vi "rigol-dg1000.vi"() -> ()   [LabVIEW 2024]
uses:
  <vilib>/Instr/_visa.llb/VISA Open Access Mode.ctl
  <vilib>/measure/NI_MABase.lvlib
panel:
  out "Ch2 Freq":dbl caption="output 1" format="%#_6pHz"
  out "CH2 Volt":dbl caption="output 1" format="%#_6pVpp"
  out "CH2 status":bool
  out "Waveform CH2":waveform(dbl)(graph)
  out "Waveform CH1":waveform(dbl)(graph)
  out "CH1 status":bool
  out "CH1 Volt":dbl caption="output 1" format="%#_6pVpp"
  out "Ch1 Freq":dbl caption="output 1" format="%#_6pHz"
  in  "stop":bool
  out "error out":errorcluster
  in  "error in (no error)":errorcluster
  in  "VISA resource name":refnum<visa-resource-name>="TCPIP0::172.16.15.122::inst0::INSTR"
  # "CH1"
  # "CH2"
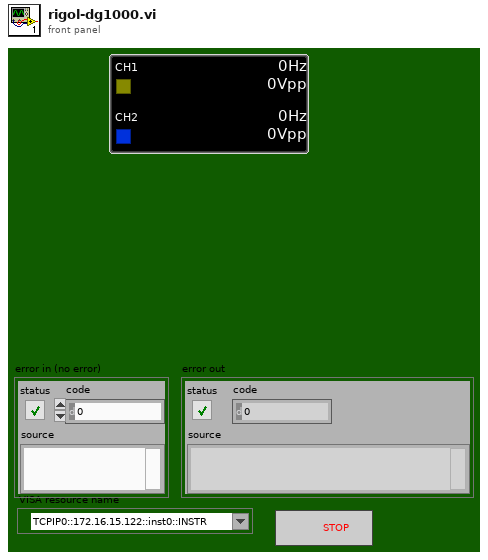
[diagram p1: front panel]
types:
  T1 = typedef "VISA Open Access Mode.ctl" = u32
  T2 = enum16{"Sine Wave", "Triangle Wave", "Square Wave", "Sawtooth Wave"}
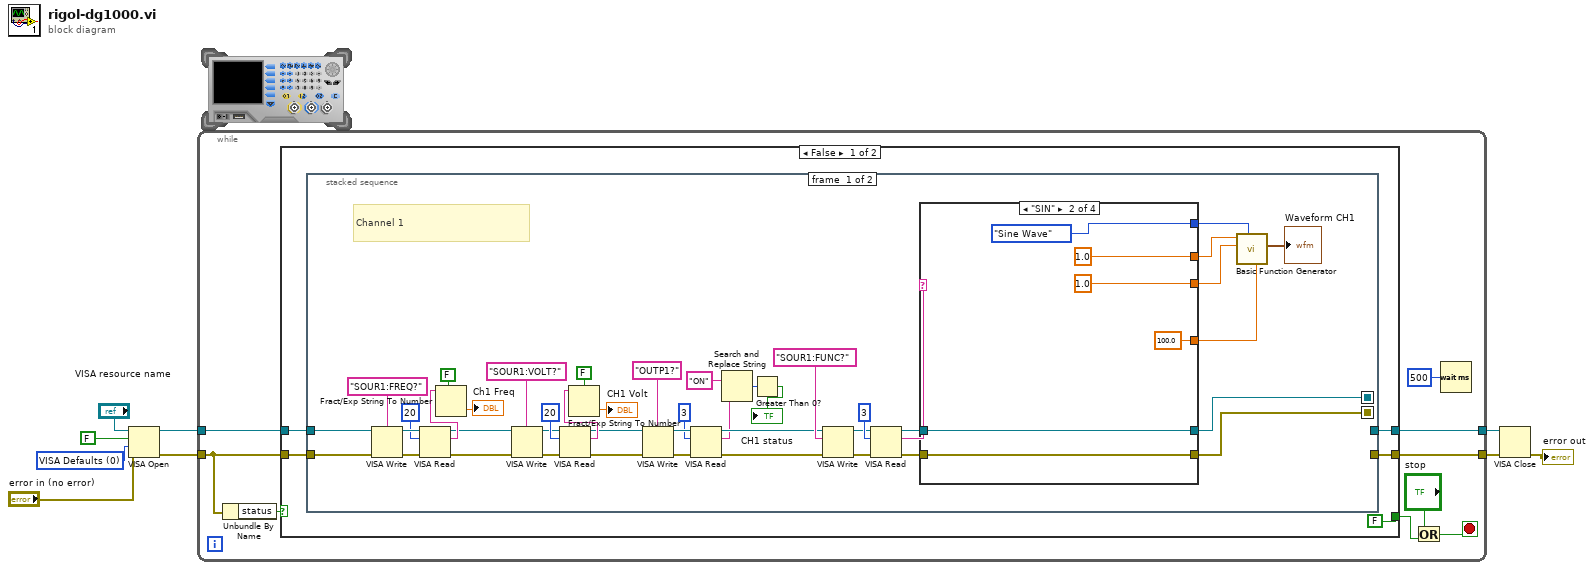
[diagram p0: block diagram]
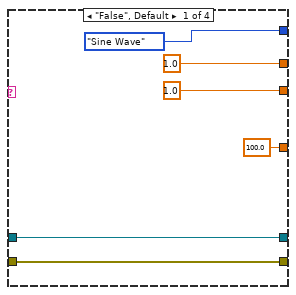
[diagram p2: hidden frame]
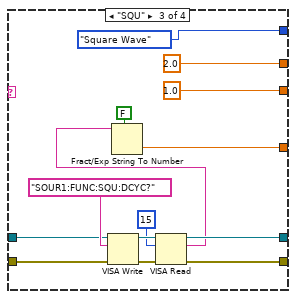
[diagram p3: hidden frame]
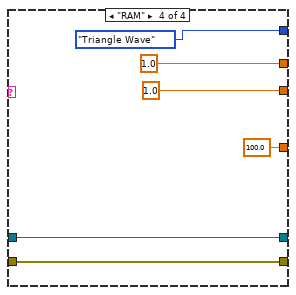
[diagram p4: hidden frame]
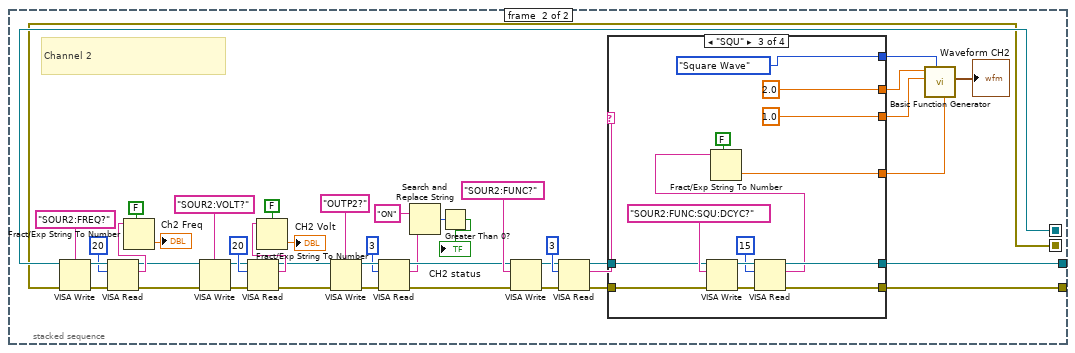
[diagram p5: hidden frame]
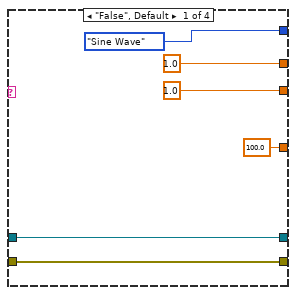
[diagram p6: hidden frame]
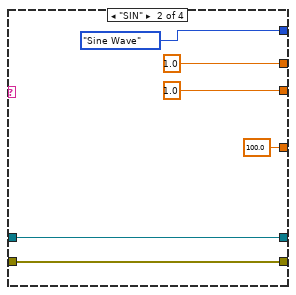
[diagram p7: hidden frame]
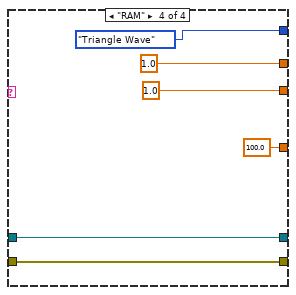
[diagram p8: hidden frame]
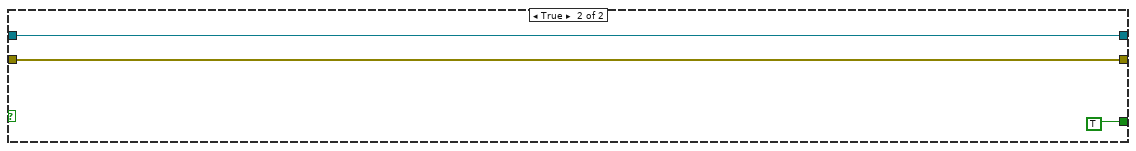
[diagram p9: hidden frame]
diagram:
  w7 = T1 0 items=["VISA Defaults"=0, "Exclusive Lock"=1, "Load Configured Settings"=4] ("Access Mode")
  n1 = VISA Open(duplicate session (F)=FALSE, access mode=w7, error in (no error)="error in (no error)", VISA resource name="VISA resource name") -> (VISA resource name=w4:refnum<visa-resource-name>, error out=w5:errorcluster)  [unwired: 1 in]
  n2 = while {
    tunnel: w5 -> [w14]
    tunnel: w4 -> [w17]
    tunnel: [w15] -> w2
    tunnel: [w16] -> w1
    stop <- w12 stop-if-true
    n3 = Unbundle By Name(w14) -> ("status"=w13:bool)
    n4 = case shown="False" w13 {
      tunnel: w17 -> [w22 w178]
      tunnel: [w21 w178] -> w16
      tunnel: [w20 w177] -> w15
      tunnel: w14 -> [w23 w177]
      tunnel: [FALSE TRUE] -> w10
      frame False {
        n5 = stacked-sequence {
          seq-local: [w25 _] -> [_ w103]
          seq-local: [w24 _] -> [_ w102]
          tunnel: w23 -> [w64 _]
          tunnel: w22 -> [w62 _]
          tunnel: [_ w101] -> w21
          tunnel: [_ w100] -> w20
          frame #0 {
            # "Channel 1"
            n6 = VISA Write(VISA resource name=w62, write buffer="SOUR1:FREQ?" ("write buffer voltage"), error in (no error)=w64) -> (VISA resource name out=w67:refnum<visa-resource-name>, error out=w66:errorcluster)  [unwired: 1 out]
            n7 = VISA Read(VISA resource name=w67, byte count=u32 20, error in (no error)=w66) -> (VISA resource name out=w48:refnum<visa-resource-name>, read buffer=w61:string, error out=w47:errorcluster)  [unwired: 1 out]
            n8 = Fract/Exp String To Number(use system decimal point (T)=FALSE, string=w61) -> (number=→"Ch1 Freq":dbl)  [unwired: 2 in, 1 out]
            n9 = VISA Write(VISA resource name=w48, write buffer="SOUR1:VOLT?" ("write buffer voltage"), error in (no error)=w47) -> (VISA resource name out=w49:refnum<visa-resource-name>, error out=w50:errorcluster)  [unwired: 1 out]
            n10 = VISA Read(VISA resource name=w49, byte count=u32 20, error in (no error)=w50) -> (VISA resource name out=w42:refnum<visa-resource-name>, read buffer=w53:string, error out=w41:errorcluster)  [unwired: 1 out]
            n11 = Fract/Exp String To Number(use system decimal point (T)=FALSE, string=w53) -> (number=→"CH1 Volt":dbl)  [unwired: 2 in, 1 out]
            n12 = VISA Write(VISA resource name=w42, write buffer="OUTP1?" ("write buffer voltage"), error in (no error)=w41) -> (VISA resource name out=w46:refnum<visa-resource-name>, error out=w45:errorcluster)  [unwired: 1 out]
            n13 = VISA Read(VISA resource name=w46, byte count=u32 3, error in (no error)=w45) -> (VISA resource name out=w40:refnum<visa-resource-name>, read buffer=w38:string, error out=w39:errorcluster)  [unwired: 1 out]
            n14 = Search and Replace String(input string=w38, search string="ON") -> (number of replacements=w36:i32)  [unwired: 6 in, 3 out]
            n15 = Greater Than 0?(x=w36) -> (x > 0?=→"CH1 status":bool)
            n16 = VISA Write(VISA resource name=w40, write buffer="SOUR1:FUNC?" ("write buffer voltage"), error in (no error)=w39) -> (VISA resource name out=w56:refnum<visa-resource-name>, error out=w57:errorcluster)  [unwired: 1 out]
            n17 = VISA Read(VISA resource name=w56, byte count=u32 3, error in (no error)=w57) -> (VISA resource name out=w29:refnum<visa-resource-name>, read buffer=w55:string, error out=w28:errorcluster)  [unwired: 1 out]
            n18 = case shown="\"SIN\"" w55 {
              tunnel: [T2."Sine Wave" ("signal type") T2."Sine Wave" ("signal type") T2."Square Wave" ("signal type") T2."Triangle Wave" ("signal type")] -> w34
              tunnel: [1.0 ("frequency") 1.0 ("frequency") 2.0 ("frequency") 1.0 ("frequency")] -> w26
              tunnel: [1.0 ("amplitude") 1.0 ("amplitude") 1.0 ("amplitude") 1.0 ("amplitude")] -> w30
              tunnel: w29 -> [w70 w76 w84 w96]
              tunnel: w28 -> [w69 w75 w83 w95]
              tunnel: [w70 w76 w86 w96] -> w25
              tunnel: [w69 w75 w85 w95] -> w24
              tunnel: [100.0 100.0 w80 100.0] -> w27
              frame "False", Default {
              }
              frame "SIN" {
              }
              frame "SQU" {
                n19 = VISA Write(VISA resource name=w84, write buffer="SOUR1:FUNC:SQU:DCYC?" ("write buffer voltage"), error in (no error)=w83) -> (VISA resource name out=w90:refnum<visa-resource-name>, error out=w89:errorcluster)  [unwired: 1 out]
                n20 = VISA Read(VISA resource name=w90, byte count=u32 15, error in (no error)=w89) -> (VISA resource name out=w86:refnum<visa-resource-name>, read buffer=w81:string, error out=w85:errorcluster)  [unwired: 1 out]
                n21 = Fract/Exp String To Number(use system decimal point (T)=FALSE, string=w81) -> (number=w80:dbl)  [unwired: 2 in, 1 out]
              }
              frame "RAM" {
              }
            }
            n22 = call <vilib>:"Basic Function Generator.vi"("square wave duty cycle (%)"=w27, "signal type"=w34, "amplitude"=w30, "frequency"=w26) -> ("signal out"=→"Waveform CH1":waveform(dbl))  [unwired: 5 in, 2 out]
          }
          frame #1 {
            # "Channel 2"
            n23 = VISA Write(VISA resource name=w103, write buffer="SOUR2:FREQ?" ("write buffer voltage"), error in (no error)=w102) -> (VISA resource name out=w143:refnum<visa-resource-name>, error out=w142:errorcluster)  [unwired: 1 out]
            n24 = VISA Read(VISA resource name=w143, byte count=u32 20, error in (no error)=w142) -> (VISA resource name out=w126:refnum<visa-resource-name>, read buffer=w139:string, error out=w125:errorcluster)  [unwired: 1 out]
            n25 = Fract/Exp String To Number(use system decimal point (T)=FALSE, string=w139) -> (number=→"Ch2 Freq":dbl)  [unwired: 2 in, 1 out]
            n26 = VISA Write(VISA resource name=w126, write buffer="SOUR2:VOLT?" ("write buffer voltage"), error in (no error)=w125) -> (VISA resource name out=w127:refnum<visa-resource-name>, error out=w128:errorcluster)  [unwired: 1 out]
            n27 = VISA Read(VISA resource name=w127, byte count=u32 20, error in (no error)=w128) -> (VISA resource name out=w120:refnum<visa-resource-name>, read buffer=w131:string, error out=w119:errorcluster)  [unwired: 1 out]
            n28 = Fract/Exp String To Number(use system decimal point (T)=FALSE, string=w131) -> (number=→"CH2 Volt":dbl)  [unwired: 2 in, 1 out]
            n29 = VISA Write(VISA resource name=w120, write buffer="OUTP2?" ("write buffer voltage"), error in (no error)=w119) -> (VISA resource name out=w124:refnum<visa-resource-name>, error out=w123:errorcluster)  [unwired: 1 out]
            n30 = VISA Read(VISA resource name=w124, byte count=u32 3, error in (no error)=w123) -> (VISA resource name out=w118:refnum<visa-resource-name>, read buffer=w116:string, error out=w117:errorcluster)  [unwired: 1 out]
            n31 = Search and Replace String(input string=w116, search string="ON") -> (number of replacements=w114:i32)  [unwired: 6 in, 3 out]
            n32 = Greater Than 0?(x=w114) -> (x > 0?=→"CH2 status":bool)
            n33 = VISA Write(VISA resource name=w118, write buffer="SOUR2:FUNC?" ("write buffer voltage"), error in (no error)=w117) -> (VISA resource name out=w134:refnum<visa-resource-name>, error out=w135:errorcluster)  [unwired: 1 out]
            n34 = VISA Read(VISA resource name=w134, byte count=u32 3, error in (no error)=w135) -> (VISA resource name out=w107:refnum<visa-resource-name>, read buffer=w133:string, error out=w106:errorcluster)  [unwired: 1 out]
            n35 = case shown="\"SQU\"" w133 {
              tunnel: [T2."Sine Wave" ("signal type") T2."Sine Wave" ("signal type") T2."Square Wave" ("signal type") T2."Triangle Wave" ("signal type")] -> w112
              tunnel: [1.0 ("frequency") 1.0 ("frequency") 2.0 ("frequency") 1.0 ("frequency")] -> w104
              tunnel: [1.0 ("amplitude") 1.0 ("amplitude") 1.0 ("amplitude") 1.0 ("amplitude")] -> w108
              tunnel: w107 -> [w146 w152 w160 w172]
              tunnel: w106 -> [w145 w151 w159 w171]
              tunnel: [w146 w152 w162 w172] -> w101
              tunnel: [w145 w151 w161 w171] -> w100
              tunnel: [100.0 100.0 w156 100.0] -> w105
              frame "False", Default {
              }
              frame "SIN" {
              }
              frame "SQU" {
                n36 = VISA Write(VISA resource name=w160, write buffer="SOUR2:FUNC:SQU:DCYC?" ("write buffer voltage"), error in (no error)=w159) -> (VISA resource name out=w166:refnum<visa-resource-name>, error out=w165:errorcluster)  [unwired: 1 out]
                n37 = VISA Read(VISA resource name=w166, byte count=u32 15, error in (no error)=w165) -> (VISA resource name out=w162:refnum<visa-resource-name>, read buffer=w157:string, error out=w161:errorcluster)  [unwired: 1 out]
                n38 = Fract/Exp String To Number(use system decimal point (T)=FALSE, string=w157) -> (number=w156:dbl)  [unwired: 2 in, 1 out]
              }
              frame "RAM" {
              }
            }
            n39 = call <vilib>:"Basic Function Generator.vi"("square wave duty cycle (%)"=w105, "signal type"=w112, "amplitude"=w108, "frequency"=w104) -> ("signal out"=→"Waveform CH2":waveform(dbl))  [unwired: 5 in, 2 out]
          }
        }
      }
      frame True {
      }
    }
    n40 = Or(x="stop", y=w10) -> (x .or. y?=w12:bool)
    n41 = Wait (ms)(milliseconds to wait=u32 500) -> ()  [unwired: 1 out]
  }
  n42 = VISA Close(VISA resource name=w1, error in (no error)=w2) -> (error out=→"error out":errorcluster)
